vi "update-image-data-on-trace.vi"(4 "detrend":bool=TRUE, 9 "iterator":i32, 10 "master-image-data-n":dbl[][](array[numeric]), 11 "avg-data-row":dbl[](array[numeric])) -> (3 "master-image-data-out":dbl[][](array[numeric]))   [LabVIEW 2017]
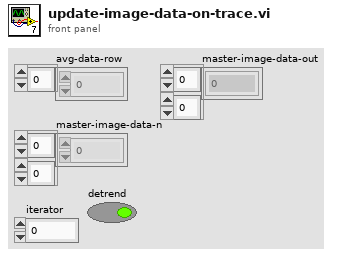
[diagram p1: front panel]
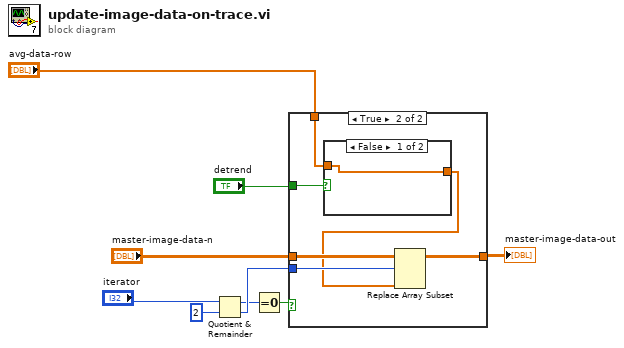
[diagram p0: block diagram]
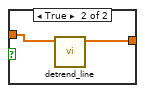
[diagram p3: hidden frame]
diagram:
  n1 = Quotient & Remainder(x="iterator", y=2) -> (x-y*floor(x/y)=w8:i32, floor(x/y)=w9:i32)
  n2 = Equal To 0?(x=w8) -> (x = 0?=w7:bool)
  n3 = case shown="True" w7 {
    tunnel: w9 -> [_ w16]
    tunnel: [w10 w15] -> w3
    tunnel: "master-image-data-n" -> [w10 w14]
    tunnel: "avg-data-row" -> [_ w13]
    tunnel: "detrend" -> [_ w11]
    frame False {
    }
    frame True {
      n4 = case shown="False" w11 {
        tunnel: w13 -> [w17 w19]
        tunnel: [w17 w18] -> w12
        frame False {
        }
        frame True {
          n5 = call "detrend_line.vi"("data_in"=w19) -> ("detrended"=w18:dbl[])  [unwired: 10 in]
        }
      }
      n6 = Replace Array Subset(array=w14, new element=w12, index (row)=w16) -> (w15:dbl[][])  [unwired: 1 in]
    }
  }
  "master-image-data-out" <- w3
